vi "24点 - LabVIEW2014 - yuanchgen.vi"() -> ()   [LabVIEW 2014]
uses:
  <vilib>/Utility/file.llb/Read From Spreadsheet File (string).vi
panel:
  out "有解次数":dbl
  in  "重做标志":bool
  in  "重做次数":i32=1
  out "错题库":dbl[][](array[numeric])
  out "time2":dbl=525974.5673637404 caption="相对秒钟" format="%_19f"
  out "time1":dbl=327.1343983679108 caption="相对秒钟" format="%_19f"
  out "time o":dbl=70.42058685328811 caption="相对秒钟" format="%_4f"
  out "开始时间":dbl=525967.1962749355 caption="相对秒钟" format="%_19f"
  out "结束时间":dbl=525974.5673695413 caption="相对秒钟" format="%_19f"
  out "新游戏标志 2":bool
  out "成功次数":dbl=1.0
  out "失败次数":dbl
  in  "新游戏标志":bool
  in  "时间计算标志":bool=TRUE
  out "所有正解":string[](array[string])=["8*(12-9/1)", "8*(12-9)*1"]
  out "算法总数":i32=2
  out "运算符输入次数":dbl
  out "牌值 4":u32=9
  out "牌值 3":u32=1
  out "牌值 2":u32=12
  out "牌值1":u32=8
  in  "游戏界面":enum32{"主界面", "批量计算"}(tab)
  in  "牌遮 3":enum32{"选项卡 1", "选项卡 2"}(tab)
  in  "批量计算":bool=TRUE
  in  "错题重做":bool
  in  "退出游戏":bool=TRUE
  out "已用时间":string="4.04s"
  out "分数提示":string="胜利/失败: 1/0"
  in  "重置":bool
  out "公式显示":string
  in  "牌遮 4":enum32{"选项卡 1", "选项卡 2"}(tab)
  in  "牌遮 2":enum32{"选项卡 1", "选项卡 2"}(tab)
  in  "牌遮 1":enum32{"选项卡 1", "选项卡 2"}(tab)
  out "扑克牌 4":u16(ring)=48
  out "扑克牌 3":u16(ring)=27
  out "扑克牌 2":u16(ring)=51
  out "扑克牌 1":u16(ring)=47
  in  "开始游戏":bool
  in  "偷看答案":bool
  in  "无解":bool
  in  "计算":bool
  in  "右括号":bool
  in  "左括号":bool
  in  "除":bool
  in  "乘":bool
  in  "减":bool
  in  "加":bool
  in  "返回主界面":bool caption="退出游戏"
  out "表格":string[][](table)
  out "结果显示":string="本次批量计算总共完成   组数据，共耗时   s。"
  in  "文件路径输入控件":path
  # "扑克24点"
  # "24点批量计算"
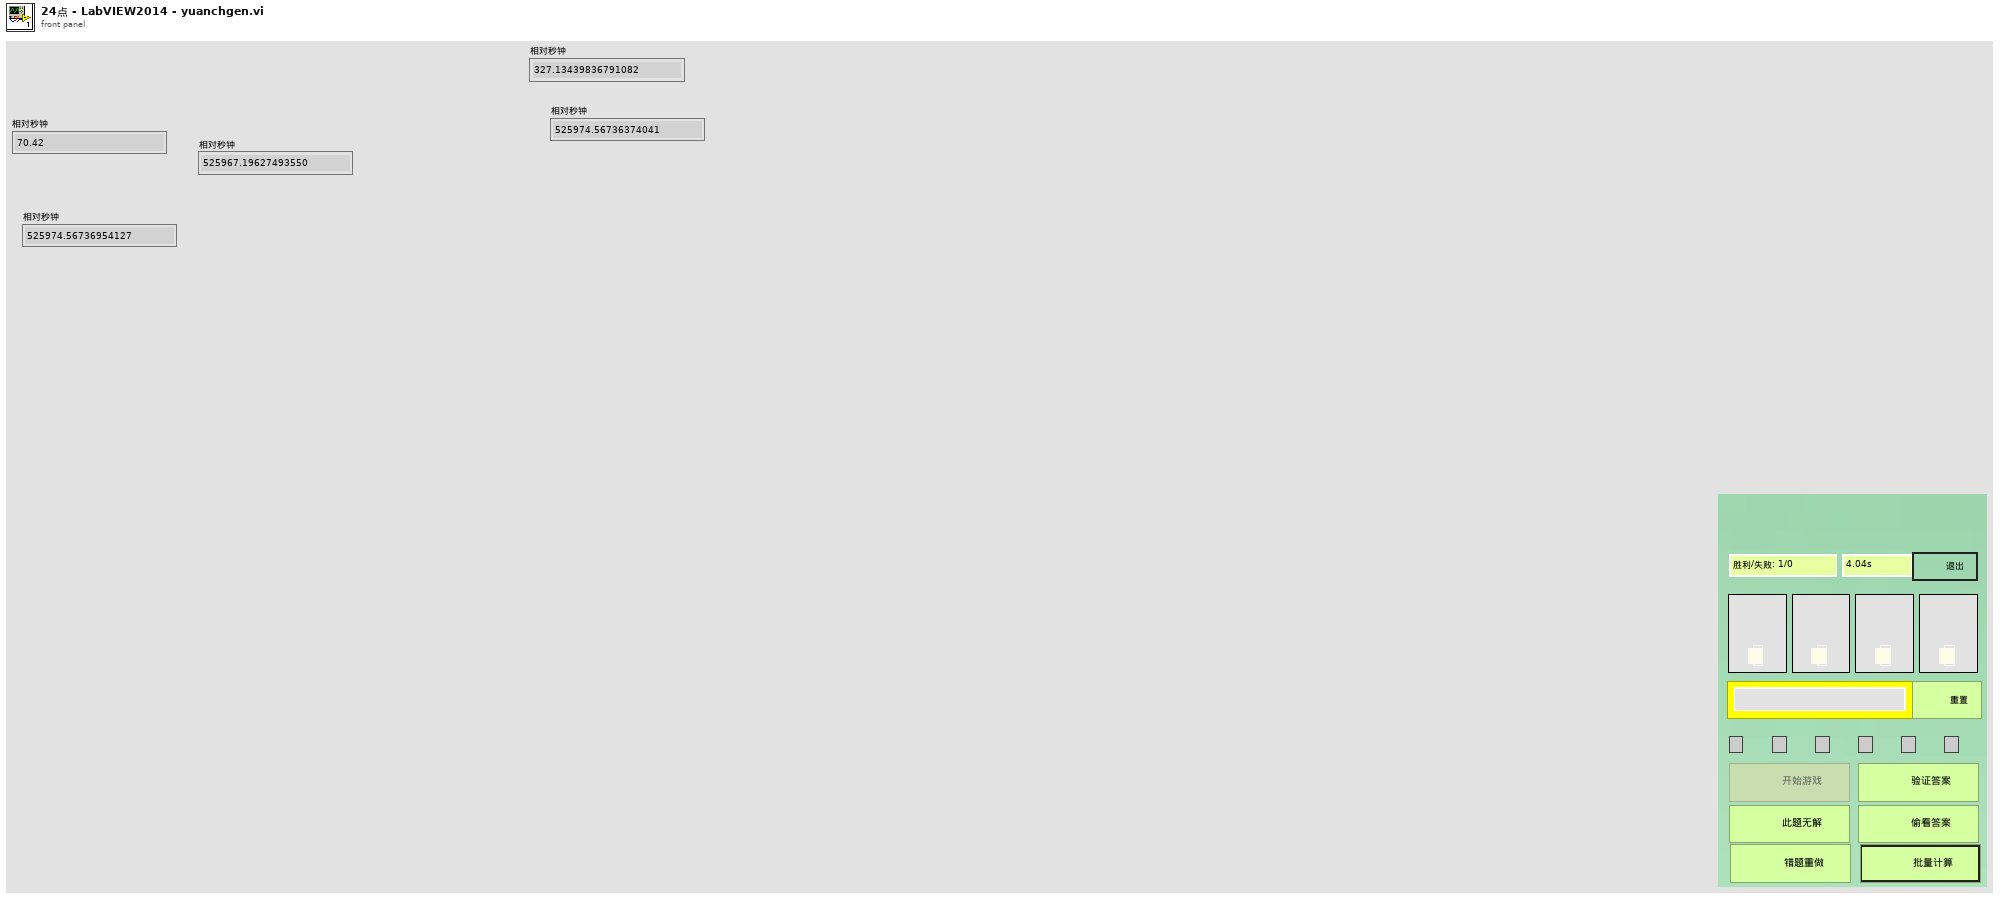
[diagram p1: front panel]
types:
  T1 = enum8{"Enabled", "Disabled", "Disabled and Grayed Out"}
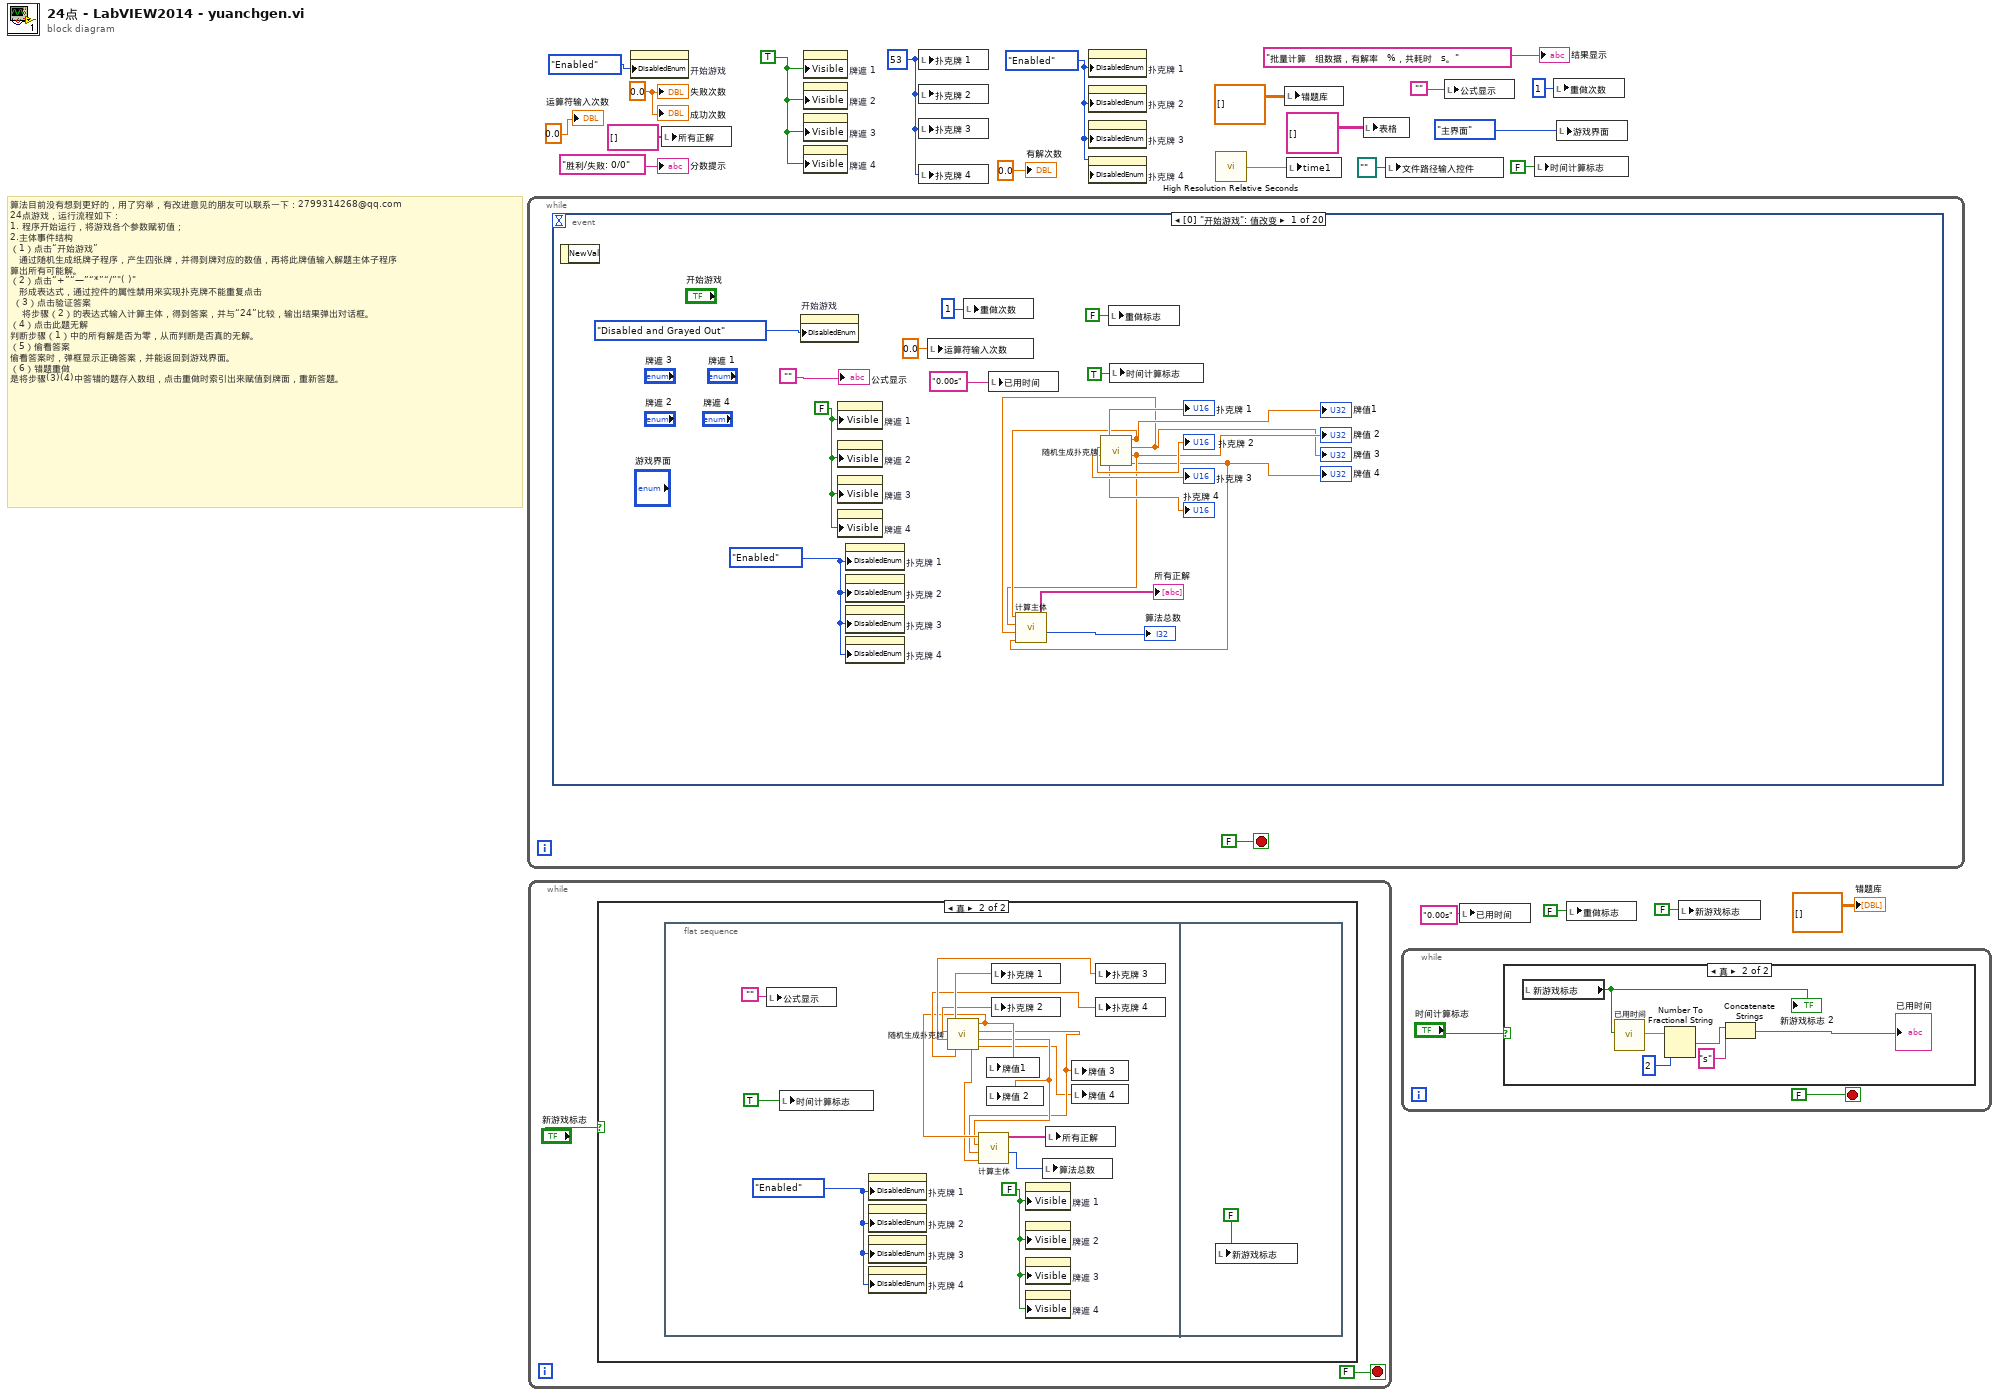
[diagram p0: block diagram]
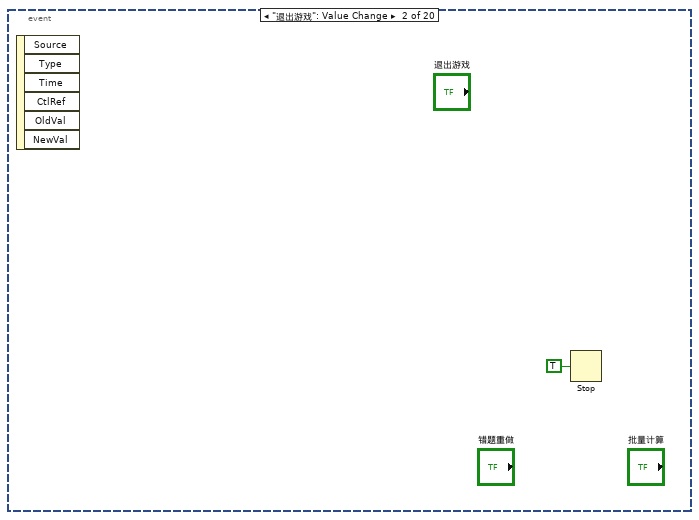
[diagram p4: hidden frame]
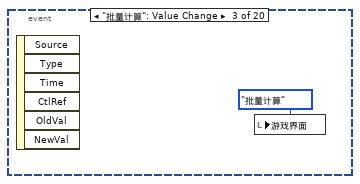
[diagram p5: hidden frame]
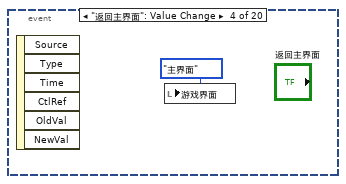
[diagram p6: hidden frame]
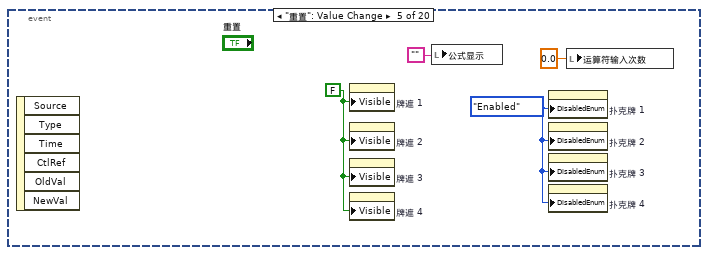
[diagram p7: hidden frame]
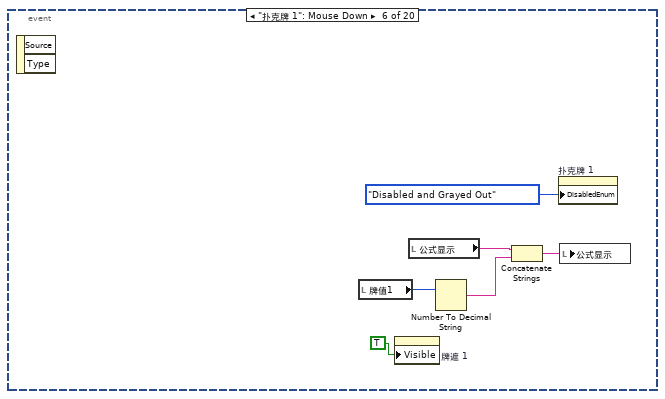
[diagram p8: hidden frame]
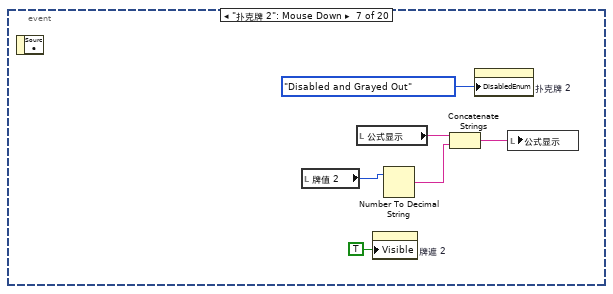
[diagram p9: hidden frame]
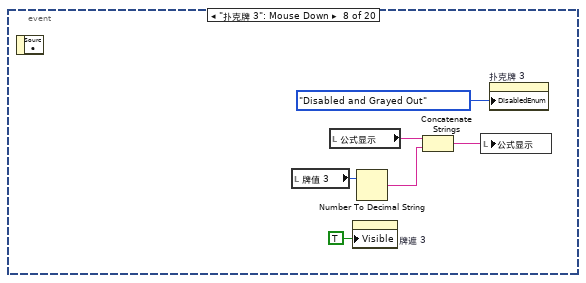
[diagram p10: hidden frame]
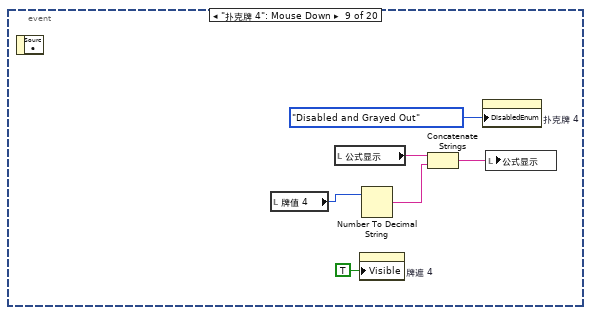
[diagram p11: hidden frame]
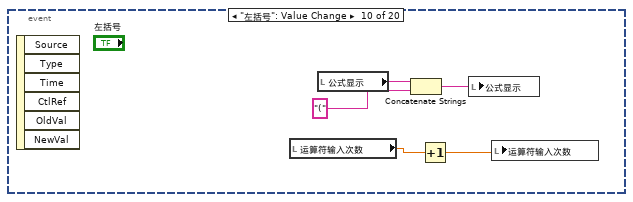
[diagram p12: hidden frame]
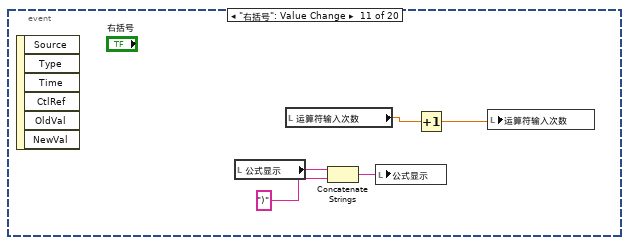
[diagram p13: hidden frame]
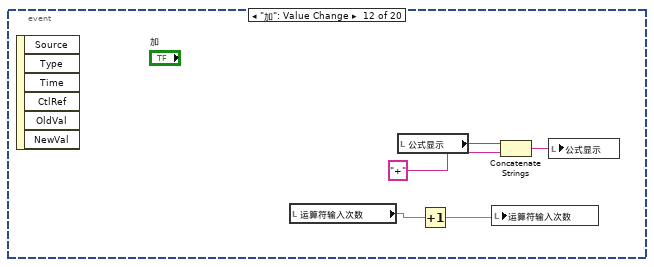
[diagram p14: hidden frame]
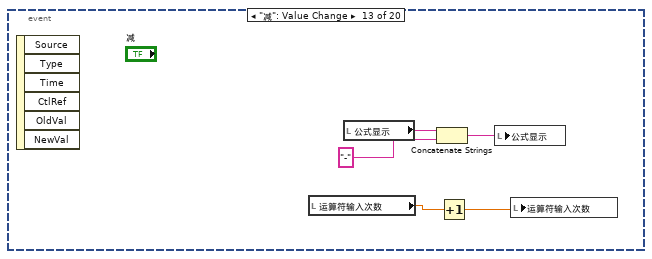
[diagram p15: hidden frame]
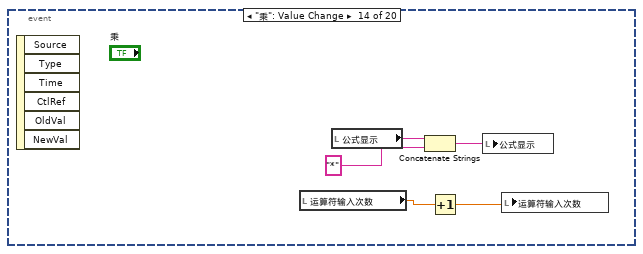
[diagram p16: hidden frame]
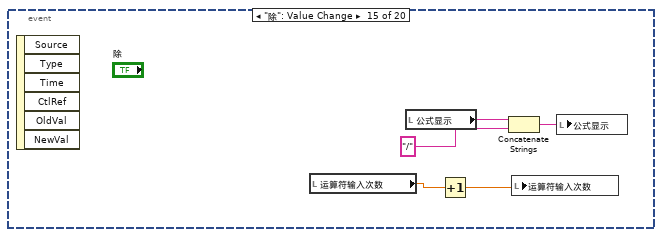
[diagram p17: hidden frame]
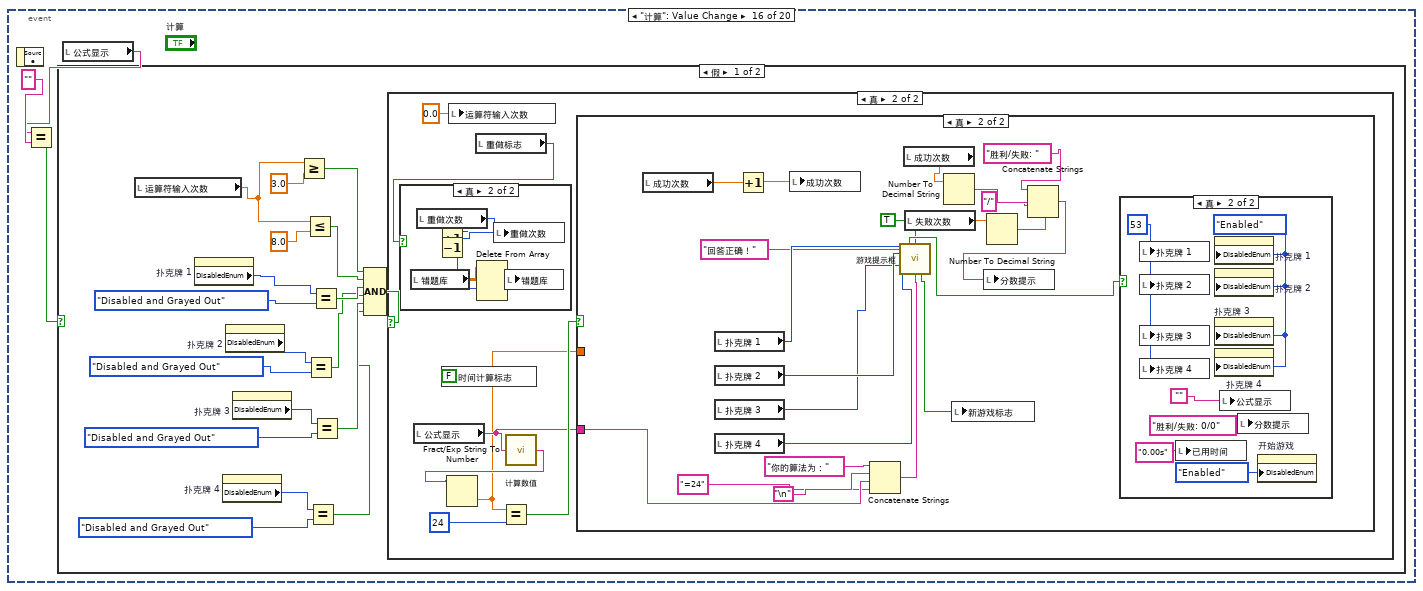
[diagram p18: hidden frame]
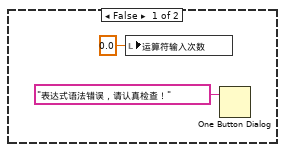
[diagram p19: hidden frame]
diagram:
  w15 = 0.0 ("运算符输入次数 2")
  w20 = TRUE ("可见")
  w21 = T1."Enabled" ("禁用")
  w22 = u16 53 ("扑克牌 1")
  # "算法目前没有想到更好的，用了穷举，有改进意见的朋友可以联系一下：2799314268@qq.com\n24点游戏，运行流程如下：\n1. 程序开始运行，将游戏各个参数赋初值；\n2.主体事件结构\n（1）点击“开始游戏”\n   通过随机生成纸牌子程序，产生四张牌，并得到牌对应的数值，再将此牌值输入解题主体子程序\n算出所有可能解。\n（2）点击“+”“—”“*”“/”\"( )\"\n   形成表达式，通过控件的属性禁用来实现扑克牌不能重复点击\n （3）点击验证答案\n    将步骤（2）的表达式输入计算主体，得到答案，并与“24”比较，输出结果弹出对话框。\n（4）点击此题无解\n判断步骤（1）中的所有解是否为零，从而判断是否真的无解。\n（5）偷看答案\n偷看答案时，弹框显示正确答案，并能返回到游戏界面。\n（6）错题重做\n是将步骤(3)(4)中答错的题存入数组，点击重做时索引出来赋值到牌面，重新答题。"
  n1 = while {
    stop <- FALSE stop-if-true
    n2 = event shown="[0] \"开始游戏\": 值改变" {
      selector: _ -> [_ _ _ _ _ _ _ _ _ _ _ _ _ _ _ _ _ _ _ _]
      dyn-events: _ -> [_ _ _ _ _ _ _ _ _ _ _ _ _ _ _ _ _ _ _ _]
      timeout: _ -> [_ _ _ _ _ _ _ _ _ _ _ _ _ _ _ _ _ _ _ _]
      event "开始游戏": Value Change {
        w40 = FALSE ("可见")
        w42 = T1."Enabled" ("禁用")
        n3 = event-data() -> ()  [unwired: 1 in, 1 out]
        n4 = property on="开始游戏" class="Bool"("DisabledEnum"=T1."Disabled and Grayed Out" ("禁用")) -> ()  [unwired: 2 in, 2 out]
        n5 = property on="牌遮 1" class="TabCtl (严格)"("Visible"=w40) -> ()  [unwired: 2 in, 2 out]
        n6 = property on="牌遮 2" class="TabCtl (严格)"("Visible"=w40) -> ()  [unwired: 2 in, 2 out]
        n7 = property on="牌遮 3" class="TabCtl (严格)"("Visible"=w40) -> ()  [unwired: 2 in, 2 out]
        n8 = property on="牌遮 4" class="TabCtl (严格)"("Visible"=w40) -> ()  [unwired: 2 in, 2 out]
        n9 = property on="扑克牌 1" class="Ring (严格)"("DisabledEnum"=w42) -> ()  [unwired: 2 in, 2 out]
        n10 = property on="扑克牌 2" class="Ring (严格)"("DisabledEnum"=w42) -> ()  [unwired: 2 in, 2 out]
        n11 = property on="扑克牌 3" class="Ring (严格)"("DisabledEnum"=w42) -> ()  [unwired: 2 in, 2 out]
        n12 = property on="扑克牌 4" class="Ring (严格)"("DisabledEnum"=w42) -> ()  [unwired: 2 in, 2 out]
        n13 = local write "运算符输入次数"(0.0 ("运算符输入次数")) -> ()
        n14 = local write "重做次数"(1 ("重做次数")) -> ()
        n15 = local write "已用时间"("0.00s" ("连接的字符串")) -> ()
        n16 = call "随机生成扑克牌.vi"() -> ("牌4值"=w24:dbl, "牌2值"=w26:dbl, "牌3值"=w25:dbl, "牌1值"=w27:dbl, "牌4"=→"扑克牌 4":dbl, "牌3"=→"扑克牌 3":dbl, "牌2"=→"扑克牌 2":dbl, "牌1"=→"扑克牌 1":dbl)
        "牌值1" <- w27
        "牌值 2" <- w26
        "牌值 3" <- w25
        "牌值 4" <- w24
        n17 = call "计算主体.vi"("d"=w24, "c"=w25, "b"=w26, "a"=w27) -> ("算法总数"=→"算法总数":i32, "所有正解"=→"所有正解":string[])  [unwired: 1 in, 1 out]
        n18 = local write "重做标志"(FALSE ("重做标志")) -> ()
        n19 = local write "时间计算标志"(TRUE ("布尔")) -> ()
        "公式显示" <- ""
      }
      event "退出游戏": Value Change {
        n20 = event-data() -> ()  [unwired: 1 in, 6 out]
        n21 = Stop(stop? (T)=TRUE ("停止？(T)")) -> ()
      }
      event "批量计算": Value Change {
        n22 = event-data() -> ()  [unwired: 1 in, 6 out]
        n23 = local write "游戏界面"(enum32{"主界面", "批量计算"}."批量计算" ("选项卡控件")) -> ()
      }
      event "返回主界面": Value Change {
        n24 = event-data() -> ()  [unwired: 1 in, 6 out]
        n25 = local write "游戏界面"(enum32{"主界面", "批量计算"}."主界面" ("选项卡控件")) -> ()
      }
      event "重置": Value Change {
        w47 = T1."Enabled" ("禁用")
        w48 = FALSE ("可见")
        n26 = event-data() -> ()  [unwired: 1 in, 6 out]
        n27 = property on="牌遮 1" class="TabCtl (严格)"("Visible"=w48) -> ()  [unwired: 2 in, 2 out]
        n28 = property on="牌遮 2" class="TabCtl (严格)"("Visible"=w48) -> ()  [unwired: 2 in, 2 out]
        n29 = property on="牌遮 3" class="TabCtl (严格)"("Visible"=w48) -> ()  [unwired: 2 in, 2 out]
        n30 = property on="牌遮 4" class="TabCtl (严格)"("Visible"=w48) -> ()  [unwired: 2 in, 2 out]
        n31 = local write "公式显示"("") -> ()
        n32 = property on="扑克牌 1" class="Ring (严格)"("DisabledEnum"=w47) -> ()  [unwired: 2 in, 2 out]
        n33 = property on="扑克牌 2" class="Ring (严格)"("DisabledEnum"=w47) -> ()  [unwired: 2 in, 2 out]
        n34 = property on="扑克牌 3" class="Ring (严格)"("DisabledEnum"=w47) -> ()  [unwired: 2 in, 2 out]
        n35 = property on="扑克牌 4" class="Ring (严格)"("DisabledEnum"=w47) -> ()  [unwired: 2 in, 2 out]
        n36 = local write "运算符输入次数"(0.0 ("运算符输入次数")) -> ()
      }
      event "扑克牌 1": Mouse Down {
        n37 = event-data() -> ()  [unwired: 1 in, 2 out]
        n38 = local read "牌值1"() -> (w54:u32)
        n39 = property on="牌遮 1" class="TabCtl (严格)"("Visible"=TRUE ("可见")) -> ()  [unwired: 2 in, 2 out]
        n40 = local read "公式显示"() -> (w52:string)
        n41 = Number To Decimal String(number=w54) -> (decimal integer string=w53:string)  [unwired: 1 in]
        n42 = Concatenate Strings(w52, w53) -> (w51:string)
        n43 = property on="扑克牌 1" class="Ring (严格)"("DisabledEnum"=T1."Disabled and Grayed Out" ("禁用")) -> ()  [unwired: 2 in, 2 out]
        n44 = local write "公式显示"(w51) -> ()
      }
      event "扑克牌 2": Mouse Down {
        n45 = event-data() -> ()  [unwired: 1 in, 1 out]
        n46 = local read "牌值 2"() -> (w57:u32)
        n47 = local read "公式显示"() -> (w59:string)
        n48 = property on="牌遮 2" class="TabCtl (严格)"("Visible"=TRUE ("可见")) -> ()  [unwired: 2 in, 2 out]
        n49 = Number To Decimal String(number=w57) -> (decimal integer string=w60:string)  [unwired: 1 in]
        n50 = Concatenate Strings(w59, w60) -> (w58:string)
        n51 = property on="扑克牌 2" class="Ring (严格)"("DisabledEnum"=T1."Disabled and Grayed Out" ("禁用")) -> ()  [unwired: 2 in, 2 out]
        n52 = local write "公式显示"(w58) -> ()
      }
      event "扑克牌 3": Mouse Down {
        n53 = event-data() -> ()  [unwired: 1 in, 1 out]
        n54 = local read "牌值 3"() -> (w63:u32)
        n55 = local read "公式显示"() -> (w66:string)
        n56 = property on="牌遮 3" class="TabCtl (严格)"("Visible"=TRUE ("可见")) -> ()  [unwired: 2 in, 2 out]
        n57 = Number To Decimal String(number=w63) -> (decimal integer string=w64:string)  [unwired: 1 in]
        n58 = Concatenate Strings(w66, w64) -> (w65:string)
        n59 = local write "公式显示"(w65) -> ()
        n60 = property on="扑克牌 3" class="Ring (严格)"("DisabledEnum"=T1."Disabled and Grayed Out" ("禁用")) -> ()  [unwired: 2 in, 2 out]
      }
      event "扑克牌 4": Mouse Down {
        n61 = event-data() -> ()  [unwired: 1 in, 1 out]
        n62 = local read "牌值 4"() -> (w69:u32)
        n63 = local read "公式显示"() -> (w72:string)
        n64 = property on="牌遮 4" class="TabCtl (严格)"("Visible"=TRUE ("可见")) -> ()  [unwired: 2 in, 2 out]
        n65 = Number To Decimal String(number=w69) -> (decimal integer string=w70:string)  [unwired: 1 in]
        n66 = Concatenate Strings(w72, w70) -> (w71:string)
        n67 = property on="扑克牌 4" class="Ring (严格)"("DisabledEnum"=T1."Disabled and Grayed Out" ("禁用")) -> ()  [unwired: 2 in, 2 out]
        n68 = local write "公式显示"(w71) -> ()
      }
      event "左括号": Value Change {
        n69 = event-data() -> ()  [unwired: 1 in, 6 out]
        n70 = local read "运算符输入次数"() -> (w75:dbl)
        n71 = local read "公式显示"() -> (w78:string)
        n72 = Concatenate Strings(w78, "(" ("字符串")) -> (w77:string)
        n73 = Increment(x=w75) -> (x+1=w74:dbl)
        n74 = local write "公式显示"(w77) -> ()
        n75 = local write "运算符输入次数"(w74) -> ()
      }
      event "右括号": Value Change {
        n76 = event-data() -> ()  [unwired: 1 in, 6 out]
        n77 = local read "公式显示"() -> (w83:string)
        n78 = local read "运算符输入次数"() -> (w80:dbl)
        n79 = Concatenate Strings(w83, ")" ("字符串")) -> (w82:string)
        n80 = local write "公式显示"(w82) -> ()
        n81 = Increment(x=w80) -> (x+1=w79:dbl)
        n82 = local write "运算符输入次数"(w79) -> ()
      }
      event "加": Value Change {
        n83 = event-data() -> ()  [unwired: 1 in, 6 out]
        n84 = local read "运算符输入次数"() -> (w85:dbl)
        n85 = local read "公式显示"() -> (w88:string)
        n86 = Increment(x=w85) -> (x+1=w84:dbl)
        n87 = local write "运算符输入次数"(w84) -> ()
        n88 = Concatenate Strings(w88, "+" ("字符串")) -> (w87:string)
        n89 = local write "公式显示"(w87) -> ()
      }
      event "减": Value Change {
        n90 = event-data() -> ()  [unwired: 1 in, 6 out]
        n91 = local read "运算符输入次数"() -> (w90:dbl)
        n92 = local read "公式显示"() -> (w93:string)
        n93 = Concatenate Strings(w93, "-" ("字符串")) -> (w92:string)
        n94 = Increment(x=w90) -> (x+1=w89:dbl)
        n95 = local write "公式显示"(w92) -> ()
        n96 = local write "运算符输入次数"(w89) -> ()
      }
      event "乘": Value Change {
        n97 = event-data() -> ()  [unwired: 1 in, 6 out]
        n98 = local read "运算符输入次数"() -> (w95:dbl)
        n99 = local read "公式显示"() -> (w98:string)
        n100 = Concatenate Strings(w98, "*" ("字符串")) -> (w97:string)
        n101 = Increment(x=w95) -> (x+1=w94:dbl)
        n102 = local write "公式显示"(w97) -> ()
        n103 = local write "运算符输入次数"(w94) -> ()
      }
      event "除": Value Change {
        n104 = event-data() -> ()  [unwired: 1 in, 6 out]
        n105 = local read "运算符输入次数"() -> (w100:dbl)
        n106 = local read "公式显示"() -> (w103:string)
        n107 = Increment(x=w100) -> (x+1=w99:dbl)
        n108 = Concatenate Strings(w103, "/" ("字符串")) -> (w102:string)
        n109 = local write "运算符输入次数"(w99) -> ()
        n110 = local write "公式显示"(w102) -> ()
      }
      event "计算": Value Change {
        n111 = event-data() -> ()  [unwired: 1 in, 1 out]
        n112 = local read "公式显示"() -> (w105:string)
        n113 = Equal?(x=w105, y="" ("公式显示")) -> (x = y?=w104:bool)
        n114 = case shown="假" w104 {
          frame False {
            n115 = local read "运算符输入次数"() -> (w108:dbl)
            n116 = property on="扑克牌 1" class="Ring (严格)"() -> ("DisabledEnum"=w109:T1)  [unwired: 2 in, 2 out]
            n117 = property on="扑克牌 4" class="Ring (严格)"() -> ("DisabledEnum"=w117:T1)  [unwired: 2 in, 2 out]
            n118 = property on="扑克牌 2" class="Ring (严格)"() -> ("DisabledEnum"=w121:T1)  [unwired: 2 in, 2 out]
            n119 = property on="扑克牌 3" class="Ring (严格)"() -> ("DisabledEnum"=w119:T1)  [unwired: 2 in, 2 out]
            n120 = Greater Or Equal?(x=w108, y=3.0) -> (x >= y?=w115:bool)
            n121 = Less Or Equal?(x=w108, y=8.0) -> (x <= y?=w107:bool)
            n122 = Equal?(x=w121, y=T1."Disabled and Grayed Out" ("禁用")) -> (x = y?=w113:bool)
            n123 = Equal?(x=w117, y=T1."Disabled and Grayed Out" ("禁用")) -> (x = y?=w111:bool)
            n124 = Equal?(x=w109, y=T1."Disabled and Grayed Out" ("禁用")) -> (x = y?=w114:bool)
            n125 = Equal?(x=w119, y=T1."Disabled and Grayed Out" ("禁用")) -> (x = y?=w112:bool)
            n126 = Compound Arithmetic op=AND(w115, w107, w114, w113, w112, w111) -> (w110:bool)
            n127 = case shown="真" w110 {
              frame False {
                n128 = local write "运算符输入次数"(0.0 ("运算符输入次数")) -> ()
                n129 = One Button Dialog(message="表达式语法错误，请认真检查！" ("消息")) -> ()  [unwired: 1 in, 1 out]
              }
              frame True {
                n130 = local read "公式显示"() -> (w131:string)
                n131 = local write "时间计算标志"(FALSE ("布尔")) -> ()
                n132 = local write "运算符输入次数"(0.0 ("运算符输入次数")) -> ()
                n133 = local read "重做标志"() -> (w128:bool)
                n134 = case shown="真" w128 {
                  frame False {
                  }
                  frame True {
                    n135 = local read "错题库"() -> (w138:dbl[][])
                    n136 = local read "重做次数"() -> (w135:i32)
                    n137 = Increment(x=w135) -> (x+1=w136:i32)
                    n138 = Decrement(x=w135) -> (x-1=w139:i32)
                    n139 = Delete From Array(array=w138, index (row)=w139) -> (array with subset deleted=w137:dbl[][])  [unwired: 2 in, 1 out]
                    n140 = local write "重做次数"(w136) -> ()
                    n141 = local write "错题库"(w137) -> ()
                  }
                }
                n142 = call "计算数值.vi"("表达式"=w131) -> ("结果"=w132:string)
                n143 = Fract/Exp String To Number(string=w132) -> (number=w130:dbl)  [unwired: 3 in, 1 out]
                n144 = Equal?(x=w130, y=24 ("x")) -> (x = y?=w133:bool)
                n145 = case shown="真" w133 {
                  tunnel: w130 -> [w149 _]
                  tunnel: w131 -> [_ w222]
                  frame False {
                    n146 = local read "成功次数"() -> (w146:dbl)
                    n147 = local read "失败次数"() -> (w142:dbl)
                    n148 = local read "所有正解"() -> (w153:string[])
                    n149 = local read "失败次数"() -> (w148:dbl)
                    n150 = Number To Decimal String(number=w146) -> (decimal integer string=w144:string)  [unwired: 1 in]
                    n151 = Array Size(array=w153) -> (size(s)=w152:i32)
                    n152 = Number To Decimal String(number=w142) -> (decimal integer string=w141:string)  [unwired: 1 in]
                    n153 = Increment(x=w148) -> (x+1=w147:dbl)
                    n154 = local write "失败次数"(w147) -> ()
                    n155 = Equal?(x=0, y=w152) -> (x = y?=w150:bool)
                    n156 = Concatenate Strings("胜利/失败: " ("分数提示"), w144, "/" ("字符串"), w141) -> (w140:string)
                    n157 = local write "分数提示"(w140) -> ()
                    n158 = case shown="真" w150 {
                      tunnel: w149 -> [w174 w199]
                      frame False {
                        n159 = local read "所有正解"() -> (w172:string[])
                        n160 = local read "扑克牌 1"() -> (w159:u16)
                        n161 = local read "扑克牌 2"() -> (w158:u16)
                        n162 = local read "扑克牌 3"() -> (w157:u16)
                        n163 = local read "扑克牌 4"() -> (w156:u16)
                        n164 = Array Size(array=w172) -> (size(s)=w171:i32)
                        n165 = Index Array(array=w172) -> (element=w166:string)  [unwired: 1 in]
                        n166 = Number To Decimal String(number=w171) -> (decimal integer string=w170:string)  [unwired: 1 in]
                        n167 = Number To Decimal String(number=w174) -> (decimal integer string=w177:string)  [unwired: 1 in]
                        n168 = Concatenate Strings("本题有" ("字符串"), w170, "解法！" ("字符串"), "\n", "例如:" ("字符串"), w166, "=24" ("字符串")) -> (w164:string)
                        n169 = Concatenate Strings("回答错误，你的答案为" ("消息"), w177, "！" ("字符串")) -> (w175:string)
                        n170 = call "游戏提示框.vi"("数值1"=w159, "再来一局可见"=TRUE, "结果"=w175, "数值2"=w158, "数值3"=w157, "数值4"=w156, "答案"=w164) -> ("指示灯 2"=w155:bool, "指示灯"=w163:bool)  [unwired: 3 in, 4 out]
                        n171 = local write "新游戏标志"(w163) -> ()
                        n172 = local read "错题库"() -> (w162:dbl[][])
                        n173 = Build Array(w159, w158, w157, w156) -> (w161:u16[])
                        n174 = Build Array (concatenate)(w161, w162) -> (w160:dbl[][])
                        n175 = local write "错题库"(w160) -> ()
                        n176 = case shown="真" w155 {
                          frame False {
                          }
                          frame True {
                            w184 = T1."Enabled" ("禁用")
                            w183 = u16 53 ("扑克牌 1")
                            n177 = local write "扑克牌 1"(w183) -> ()
                            n178 = local write "扑克牌 2"(w183) -> ()
                            n179 = local write "扑克牌 3"(w183) -> ()
                            n180 = local write "扑克牌 4"(w183) -> ()
                            n181 = local write "已用时间"("0.00s" ("连接的字符串")) -> ()
                            n182 = property on="扑克牌 1" class="Ring (严格)"("DisabledEnum"=w184) -> ()  [unwired: 2 in, 2 out]
                            n183 = property on="扑克牌 2" class="Ring (严格)"("DisabledEnum"=w184) -> ()  [unwired: 2 in, 2 out]
                            n184 = property on="扑克牌 3" class="Ring (严格)"("DisabledEnum"=w184) -> ()  [unwired: 2 in, 2 out]
                            n185 = property on="扑克牌 4" class="Ring (严格)"("DisabledEnum"=w184) -> ()  [unwired: 2 in, 2 out]
                            n186 = local write "公式显示"("") -> ()
                            n187 = local write "分数提示"("胜利/失败: 0/0" ("分数提示")) -> ()
                            n188 = property on="开始游戏" class="Bool"("DisabledEnum"=T1."Enabled" ("禁用")) -> ()  [unwired: 2 in, 2 out]
                          }
                        }
                      }
                      frame True {
                        n189 = local read "错题库"() -> (w191:dbl[][])
                        n190 = local read "扑克牌 1"() -> (w190:u16)
                        n191 = local read "扑克牌 2"() -> (w189:u16)
                        n192 = local read "扑克牌 3"() -> (w188:u16)
                        n193 = local read "扑克牌 4"() -> (w187:u16)
                        n194 = Build Array(w190, w189, w188, w187) -> (w192:u16[])
                        n195 = Number To Decimal String(number=w199) -> (decimal integer string=w198:string)  [unwired: 1 in]
                        n196 = Build Array (concatenate)(w192, w191) -> (w193:dbl[][])
                        n197 = local write "错题库"(w193) -> ()
                        n198 = Concatenate Strings("回答错误，你的答案为：" ("消息"), w198, "！" ("字符串")) -> (w196:string)
                        n199 = call "游戏提示框.vi"("数值1"=w190, "再来一局可见"=TRUE, "结果"=w196, "数值2"=w189, "数值3"=w188, "数值4"=w187, "答案"="正确答案：本题无解！") -> ("指示灯 2"=w186:bool, "指示灯"=w194:bool)  [unwired: 3 in, 4 out]
                        n200 = local write "新游戏标志"(w194) -> ()
                        n201 = case shown="真" w186 {
                          frame False {
                          }
                          frame True {
                            w206 = T1."Enabled" ("禁用")
                            w205 = u16 53 ("扑克牌 1")
                            n202 = local write "扑克牌 1"(w205) -> ()
                            n203 = local write "扑克牌 2"(w205) -> ()
                            n204 = local write "扑克牌 3"(w205) -> ()
                            n205 = local write "扑克牌 4"(w205) -> ()
                            n206 = local write "已用时间"("0.00s" ("连接的字符串")) -> ()
                            n207 = property on="扑克牌 1" class="Ring (严格)"("DisabledEnum"=w206) -> ()  [unwired: 2 in, 2 out]
                            n208 = property on="扑克牌 2" class="Ring (严格)"("DisabledEnum"=w206) -> ()  [unwired: 2 in, 2 out]
                            n209 = property on="扑克牌 3" class="Ring (严格)"("DisabledEnum"=w206) -> ()  [unwired: 2 in, 2 out]
                            n210 = property on="扑克牌 4" class="Ring (严格)"("DisabledEnum"=w206) -> ()  [unwired: 2 in, 2 out]
                            n211 = local write "公式显示"("") -> ()
                            n212 = local write "分数提示"("胜利/失败: 0/0" ("分数提示")) -> ()
                            n213 = property on="开始游戏" class="Bool"("DisabledEnum"=T1."Enabled" ("禁用")) -> ()  [unwired: 2 in, 2 out]
                          }
                        }
                      }
                    }
                  }
                  frame True {
                    n214 = local read "成功次数"() -> (w217:dbl)
                    n215 = local read "扑克牌 1"() -> (w228:u16)
                    n216 = local read "扑克牌 2"() -> (w227:u16)
                    n217 = local read "扑克牌 3"() -> (w226:u16)
                    n218 = local read "扑克牌 4"() -> (w225:u16)
                    n219 = Increment(x=w217) -> (x+1=w216:dbl)
                    n220 = local write "成功次数"(w216) -> ()
                    n221 = Concatenate Strings("你的算法为：" ("消息"), "\n", w222, "=24" ("字符串")) -> (w220:string)
                    n222 = call "游戏提示框.vi"("数值1"=w228, "再来一局可见"=TRUE, "结果"="回答正确！" ("消息"), "数值2"=w227, "数值3"=w226, "数值4"=w225, "答案"=w220) -> ("指示灯 2"=w208:bool, "指示灯"=w218:bool)  [unwired: 3 in, 4 out]
                    n223 = local read "成功次数"() -> (w215:dbl)
                    n224 = local read "失败次数"() -> (w212:dbl)
                    n225 = Number To Decimal String(number=w215) -> (decimal integer string=w214:string)  [unwired: 1 in]
                    n226 = local write "新游戏标志"(w218) -> ()
                    n227 = Number To Decimal String(number=w212) -> (decimal integer string=w211:string)  [unwired: 1 in]
                    n228 = Concatenate Strings("胜利/失败: " ("分数提示"), w214, "/" ("字符串"), w211) -> (w209:string)
                    n229 = local write "分数提示"(w209) -> ()
                    n230 = case shown="真" w208 {
                      frame False {
                      }
                      frame True {
                        w234 = T1."Enabled" ("禁用")
                        w233 = u16 53 ("扑克牌 1")
                        n231 = local write "扑克牌 1"(w233) -> ()
                        n232 = local write "扑克牌 2"(w233) -> ()
                        n233 = local write "扑克牌 3"(w233) -> ()
                        n234 = local write "扑克牌 4"(w233) -> ()
                        n235 = local write "已用时间"("0.00s" ("连接的字符串")) -> ()
                        n236 = property on="扑克牌 1" class="Ring (严格)"("DisabledEnum"=w234) -> ()  [unwired: 2 in, 2 out]
                        n237 = property on="扑克牌 2" class="Ring (严格)"("DisabledEnum"=w234) -> ()  [unwired: 2 in, 2 out]
                        n238 = property on="扑克牌 3" class="Ring (严格)"("DisabledEnum"=w234) -> ()  [unwired: 2 in, 2 out]
                        n239 = property on="扑克牌 4" class="Ring (严格)"("DisabledEnum"=w234) -> ()  [unwired: 2 in, 2 out]
                        n240 = local write "公式显示"("") -> ()
                        n241 = local write "分数提示"("胜利/失败: 0/0" ("分数提示")) -> ()
                        n242 = property on="开始游戏" class="Bool"("DisabledEnum"=T1."Enabled" ("禁用")) -> ()  [unwired: 2 in, 2 out]
                      }
                    }
                  }
                }
              }
            }
          }
          frame True {
            n243 = One Button Dialog(message="表达式不能为空！" ("消息")) -> ()  [unwired: 1 in, 1 out]
          }
        }
      }
      event "无解": Value Change {
        n244 = event-data() -> ()  [unwired: 1 in, 1 out]
        n245 = local read "扑克牌 1"() -> (w238:u16)
        n246 = Equal?(x=w238, y=u16 53 ("扑克牌 1")) -> (x = y?=w236:bool)
        n247 = case shown="假" w236 {
          frame False {
            n248 = local read "所有正解"() -> (w243:string[])
            n249 = Array Size(array=w243) -> (size(s)=w242:i32)
            n250 = local write "时间计算标志"(FALSE ("布尔")) -> ()
            n251 = Equal?(x=0, y=w242) -> (x = y?=w240:bool)
            n252 = case shown="假" w240 {
              frame False {
                n253 = local read "所有正解"() -> (w272:string[])
                n254 = Array Size(array=w272) -> (size(s)=w271:i32)
                n255 = Index Array(array=w272) -> (element=w266:string)  [unwired: 1 in]
                n256 = Number To Decimal String(number=w271) -> (decimal integer string=w270:string)  [unwired: 1 in]
                n257 = local read "失败次数"() -> (w262:dbl)
                n258 = local read "扑克牌 1"() -> (w251:u16)
                n259 = local read "扑克牌 2"() -> (w250:u16)
                n260 = local read "扑克牌 3"() -> (w249:u16)
                n261 = local read "扑克牌 4"() -> (w248:u16)
                n262 = Increment(x=w262) -> (x+1=w261:dbl)
                n263 = local write "失败次数"(w261) -> ()
                n264 = Concatenate Strings("本题有" ("字符串"), w270, "解法！" ("字符串"), "\n", "例如:" ("字符串"), w266, "=24" ("字符串")) -> (w265:string)
                n265 = local read "重做标志"() -> (w246:bool)
                n266 = call "游戏提示框.vi"("数值1"=w251, "再来一局可见"=TRUE, "结果"="回答错误！", "数值2"=w250, "数值3"=w249, "数值4"=w248, "答案"=w265) -> ("指示灯 2"=w245:bool, "指示灯"=w263:bool)  [unwired: 3 in, 4 out]
                n267 = case shown="真" w246 {
                  frame False {
                  }
                  frame True {
                    n268 = local read "错题库"() -> (w284:dbl[][])
                    n269 = local read "重做次数"() -> (w283:i32)
                    n270 = Decrement(x=w283) -> (x-1=w285:i32)
                    n271 = Delete From Array(array=w284, index (row)=w285) -> (array with subset deleted=w281:dbl[][])  [unwired: 2 in, 1 out]
                    n272 = Increment(x=w283) -> (x+1=w282:i32)
                    n273 = local write "重做次数"(w282) -> ()
                    n274 = local write "错题库"(w281) -> ()
                  }
                }
                n275 = local write "新游戏标志"(w263) -> ()
                n276 = local read "成功次数"() -> (w254:dbl)
                n277 = local read "失败次数"() -> (w258:dbl)
                n278 = local read "错题库"() -> (w247:dbl[][])
                n279 = Build Array(w251, w250, w249, w248) -> (w252:u16[])
                n280 = Number To Decimal String(number=w254) -> (decimal integer string=w260:string)  [unwired: 1 in]
                n281 = Build Array (concatenate)(w252, w247) -> (w253:dbl[][])
                n282 = Number To Decimal String(number=w258) -> (decimal integer string=w257:string)  [unwired: 1 in]
                n283 = local write "错题库"(w253) -> ()
                n284 = Concatenate Strings("胜利/失败: " ("分数提示"), w260, "/" ("字符串"), w257) -> (w255:string)
                n285 = local write "分数提示"(w255) -> ()
                n286 = case shown="真" w245 {
                  frame False {
                  }
                  frame True {
                    w280 = T1."Enabled" ("禁用")
                    w279 = u16 53 ("扑克牌 1")
                    n287 = local write "扑克牌 1"(w279) -> ()
                    n288 = local write "扑克牌 2"(w279) -> ()
                    n289 = local write "扑克牌 3"(w279) -> ()
                    n290 = local write "扑克牌 4"(w279) -> ()
                    n291 = local write "已用时间"("0.00s" ("连接的字符串")) -> ()
                    n292 = property on="扑克牌 1" class="Ring (严格)"("DisabledEnum"=w280) -> ()  [unwired: 2 in, 2 out]
                    n293 = property on="扑克牌 2" class="Ring (严格)"("DisabledEnum"=w280) -> ()  [unwired: 2 in, 2 out]
                    n294 = property on="扑克牌 3" class="Ring (严格)"("DisabledEnum"=w280) -> ()  [unwired: 2 in, 2 out]
                    n295 = property on="扑克牌 4" class="Ring (严格)"("DisabledEnum"=w280) -> ()  [unwired: 2 in, 2 out]
                    n296 = local write "公式显示"("") -> ()
                    n297 = local write "分数提示"("胜利/失败: 0/0" ("分数提示")) -> ()
                    n298 = property on="开始游戏" class="Bool"("DisabledEnum"=T1."Enabled" ("禁用")) -> ()  [unwired: 2 in, 2 out]
                  }
                }
              }
              frame True {
                n299 = local read "扑克牌 1"() -> (w302:u16)
                n300 = local read "扑克牌 2"() -> (w301:u16)
                n301 = local read "扑克牌 3"() -> (w300:u16)
                n302 = local read "扑克牌 4"() -> (w299:u16)
                n303 = local read "成功次数"() -> (w297:dbl)
                n304 = Increment(x=w297) -> (x+1=w296:dbl)
                n305 = local write "成功次数"(w296) -> ()
                n306 = call "游戏提示框.vi"("数值1"=w302, "再来一局可见"=TRUE, "结果"="回答正确！" ("消息"), "数值2"=w301, "数值3"=w300, "数值4"=w299, "答案"="本题无解！") -> ("指示灯 2"=w287:bool, "指示灯"=w298:bool)  [unwired: 3 in, 4 out]
                n307 = local read "成功次数"() -> (w289:dbl)
                n308 = local read "失败次数"() -> (w293:dbl)
                n309 = Number To Decimal String(number=w289) -> (decimal integer string=w295:string)  [unwired: 1 in]
                n310 = case shown="真" "重做标志" {
                  frame False {
                  }
                  frame True {
                    n311 = local read "错题库"() -> (w314:dbl[][])
                    n312 = local read "重做次数"() -> (w313:i32)
                    n313 = Decrement(x=w313) -> (x-1=w315:i32)
                    n314 = Delete From Array(array=w314, index (row)=w315) -> (array with subset deleted=w311:dbl[][])  [unwired: 2 in, 1 out]
                    n315 = Increment(x=w313) -> (x+1=w312:i32)
                    n316 = local write "重做次数"(w312) -> ()
                    n317 = local write "错题库"(w311) -> ()
                  }
                }
                n318 = local write "新游戏标志"(w298) -> ()
                n319 = Number To Decimal String(number=w293) -> (decimal integer string=w292:string)  [unwired: 1 in]
                n320 = Concatenate Strings("胜利/失败: " ("分数提示"), w295, "/" ("字符串"), w292) -> (w290:string)
                n321 = local write "分数提示"(w290) -> ()
                n322 = case shown="真" w287 {
                  frame False {
                  }
                  frame True {
                    w310 = T1."Enabled" ("禁用")
                    w309 = u16 53 ("扑克牌 1")
                    n323 = local write "扑克牌 1"(w309) -> ()
                    n324 = local write "扑克牌 2"(w309) -> ()
                    n325 = local write "扑克牌 3"(w309) -> ()
                    n326 = local write "扑克牌 4"(w309) -> ()
                    n327 = local write "已用时间"("0.00s" ("连接的字符串")) -> ()
                    n328 = property on="扑克牌 1" class="Ring (严格)"("DisabledEnum"=w310) -> ()  [unwired: 2 in, 2 out]
                    n329 = property on="扑克牌 2" class="Ring (严格)"("DisabledEnum"=w310) -> ()  [unwired: 2 in, 2 out]
                    n330 = property on="扑克牌 3" class="Ring (严格)"("DisabledEnum"=w310) -> ()  [unwired: 2 in, 2 out]
                    n331 = property on="扑克牌 4" class="Ring (严格)"("DisabledEnum"=w310) -> ()  [unwired: 2 in, 2 out]
                    n332 = local write "公式显示"("") -> ()
                    n333 = local write "分数提示"("胜利/失败: 0/0" ("分数提示")) -> ()
                    n334 = property on="开始游戏" class="Bool"("DisabledEnum"=T1."Enabled" ("禁用")) -> ()  [unwired: 2 in, 2 out]
                  }
                }
              }
            }
          }
          frame True {
            n335 = One Button Dialog(message="请先翻拍！" ("消息")) -> ()  [unwired: 1 in, 1 out]
          }
        }
      }
      event "偷看答案": Value Change {
        n336 = event-data() -> ()  [unwired: 1 in, 1 out]
        n337 = local read "扑克牌 1"() -> (w319:u16)
        n338 = Equal?(x=w319, y=u16 53 ("扑克牌 1")) -> (x = y?=w317:bool)
        n339 = case shown="假" w317 {
          frame False {
            n340 = local read "所有正解"() -> (w324:string[])
            n341 = local write "时间计算标志"(FALSE ("布尔")) -> ()
            n342 = Array Size(array=w324) -> (size(s)=w323:i32)
            n343 = Equal?(x=0, y=w323) -> (x = y?=w321:bool)
            n344 = case shown="真" w321 {
              frame False {
                n345 = local read "所有正解"() -> (w341:string[])
                n346 = Array Size(array=w341) -> (size(s)=w340:i32)
                n347 = Index Array(array=w341) -> (element=w335:string)  [unwired: 1 in]
                n348 = Number To Decimal String(number=w340) -> (decimal integer string=w339:string)  [unwired: 1 in]
                n349 = local read "扑克牌 1"() -> (w333:u16)
                n350 = local read "扑克牌 2"() -> (w332:u16)
                n351 = local read "扑克牌 3"() -> (w331:u16)
                n352 = local read "扑克牌 4"() -> (w330:u16)
                n353 = Concatenate Strings("本题有" ("字符串"), w339, "解法！" ("字符串"), "\n", "例如:" ("字符串"), w335, "=24" ("字符串")) -> (w334:string)
                n354 = call "游戏提示框.vi"("数值1"=w333, "结果"="此题尚未作答！", "数值2"=w332, "数值3"=w331, "数值4"=w330, "返回游戏可见"=TRUE, "答案"=w334) -> ("指示灯 2"=w326:bool, "指示灯"=w328:bool)  [unwired: 3 in, 4 out]
                n355 = local write "新游戏标志"(w328) -> ()
                n356 = case shown="真" w326 {
                  frame False {
                  }
                  frame True {
                    w348 = T1."Enabled" ("禁用")
                    w347 = u16 53 ("扑克牌 1")
                    n357 = local write "扑克牌 1"(w347) -> ()
                    n358 = local write "扑克牌 2"(w347) -> ()
                    n359 = local write "扑克牌 3"(w347) -> ()
                    n360 = local write "扑克牌 4"(w347) -> ()
                    n361 = local write "已用时间"("0.00s" ("连接的字符串")) -> ()
                    n362 = property on="扑克牌 1" class="Ring (严格)"("DisabledEnum"=w348) -> ()  [unwired: 2 in, 2 out]
                    n363 = property on="扑克牌 2" class="Ring (严格)"("DisabledEnum"=w348) -> ()  [unwired: 2 in, 2 out]
                    n364 = property on="扑克牌 3" class="Ring (严格)"("DisabledEnum"=w348) -> ()  [unwired: 2 in, 2 out]
                    n365 = property on="扑克牌 4" class="Ring (严格)"("DisabledEnum"=w348) -> ()  [unwired: 2 in, 2 out]
                    n366 = local write "公式显示"("") -> ()
                    n367 = local write "分数提示"("胜利/失败: 0/0" ("分数提示")) -> ()
                    n368 = property on="开始游戏" class="Bool"("DisabledEnum"=T1."Enabled" ("禁用")) -> ()  [unwired: 2 in, 2 out]
                  }
                }
              }
              frame True {
                n369 = local read "扑克牌 1"() -> (w356:u16)
                n370 = local read "扑克牌 2"() -> (w355:u16)
                n371 = local read "扑克牌 3"() -> (w354:u16)
                n372 = local read "扑克牌 4"() -> (w352:u16)
                n373 = call "游戏提示框.vi"("数值1"=w356, "结果"="此题尚未作答\n本题无解！" ("消息"), "数值2"=w355, "数值3"=w354, "数值4"=w352, "返回游戏可见"=TRUE) -> ("指示灯 2"=w349:bool, "指示灯"=w351:bool)  [unwired: 4 in, 4 out]
                n374 = local write "新游戏标志"(w351) -> ()
                n375 = case shown="真" w349 {
                  frame False {
                  }
                  frame True {
                    w362 = T1."Enabled" ("禁用")
                    w361 = u16 53 ("扑克牌 1")
                    n376 = local write "扑克牌 1"(w361) -> ()
                    n377 = local write "扑克牌 2"(w361) -> ()
                    n378 = local write "扑克牌 3"(w361) -> ()
                    n379 = local write "扑克牌 4"(w361) -> ()
                    n380 = local write "已用时间"("0.00s" ("连接的字符串")) -> ()
                    n381 = property on="扑克牌 1" class="Ring (严格)"("DisabledEnum"=w362) -> ()  [unwired: 2 in, 2 out]
                    n382 = property on="扑克牌 2" class="Ring (严格)"("DisabledEnum"=w362) -> ()  [unwired: 2 in, 2 out]
                    n383 = property on="扑克牌 3" class="Ring (严格)"("DisabledEnum"=w362) -> ()  [unwired: 2 in, 2 out]
                    n384 = property on="扑克牌 4" class="Ring (严格)"("DisabledEnum"=w362) -> ()  [unwired: 2 in, 2 out]
                    n385 = local write "公式显示"("") -> ()
                    n386 = local write "分数提示"("胜利/失败: 0/0" ("分数提示")) -> ()
                    n387 = property on="开始游戏" class="Bool"("DisabledEnum"=T1."Enabled" ("禁用")) -> ()  [unwired: 2 in, 2 out]
                  }
                }
              }
            }
          }
          frame True {
            n388 = One Button Dialog(message="请先翻拍！" ("消息")) -> ()  [unwired: 1 in, 1 out]
          }
        }
      }
      event "文件路径输入控件": Value Change {
        n389 = event-data() -> ()  [unwired: 1 in, 1 out]
        n390 = call-poly <vilib>:"Read From Spreadsheet File.vi"("file path (dialog if empty)"="文件路径输入控件") -> ("all rows"=w370:string[][])  [unwired: 6 in, 4 out]
        n391 = local write "结果显示"("批量计算   组数据，有解率   %，共耗时   s。" ("字符串")) -> ()
        n392 = local write "表格"(string[][] [] ("表格")) -> ()
        n393 = local write "有解次数"(0.0 ("无解次数")) -> ()
        n394 = Array Size(array=w370) -> (size(s)=w368:i32[])
        n395 = Index Array(array=w368) -> (element=w369:i32)  [unwired: 1 in]
        n396 = for {
          N: w369 -> [w371]
          tunnel: w370 -> [w387] mode=indexing
          i -> [w376]
          n397 = Quotient & Remainder(x=w376, y=2) -> (x-y*floor(x/y)=w400:i32)  [unwired: 1 out]
          n398 = Index Array(array=w387) -> (element=w374:string)  [unwired: 1 in]
          n399 = Equal?(x=w376, y=0) -> (x = y?=w393:bool)
          n400 = Decrement(x=w371) -> (x-1=w382:i32)
          n401 = Equal?(x=w400, y=1) -> (x = y?=w402:bool)
          n402 = Match Pattern(string=w374, regular expression="," ("正则表达式")) -> (before substring=w412:string, after substring=w417:string)  [unwired: 1 in, 2 out]
          n403 = Select(t=TRUE, s=w402, f=FALSE) -> (s? t:f=w383:bool)
          n404 = Equal?(x=w376, y=w382) -> (x = y?=w392:bool)
          n405 = Decimal String To Number(string=w412) -> (number=w381:i32)  [unwired: 2 in, 1 out]
          n406 = case shown="真" w392 {
            selector: w392 -> [_ w419]
            tunnel: [_ w419] -> w372
            frame False {
            }
            frame True {
              n407 = call <vilib>:"High Resolution Relative Seconds.vi"() -> ("relative seconds"=→"结束时间":dbl)
            }
          }
          n408 = case shown="真" w393 {
            frame False {
            }
            frame True {
              n409 = call <vilib>:"High Resolution Relative Seconds.vi"() -> ("relative seconds"=→"开始时间":dbl)
            }
          }
          n410 = case shown="真" w383 {
            frame False {
              n411 = call <vilib>:"High Resolution Relative Seconds.vi"() -> ("relative seconds"=w442:dbl)
              "time1" <- w442
              n412 = local read "time2"() -> (w447:dbl)
              n413 = Subtract(x=w447, y=w442) -> (x-y=w446:dbl)
              n414 = Absolute Value(x=w446) -> (abs(x)=w445:dbl)
              n415 = Multiply(x=w445, y=1000.0) -> (x*y=→"time o":dbl)
            }
            frame True {
              n416 = call <vilib>:"High Resolution Relative Seconds.vi"() -> ("relative seconds"=w448:dbl)
              "time2" <- w448
              n417 = local read "time1"() -> (w453:dbl)
              n418 = Subtract(x=w453, y=w448) -> (x-y=w452:dbl)
              n419 = Absolute Value(x=w452) -> (abs(x)=w451:dbl)
              n420 = Multiply(x=w451, y=1000.0) -> (x*y=w449:dbl)
              n421 = local write "time o"(w449) -> ()
            }
          }
          n422 = Match Pattern(string=w417, regular expression="," ("正则表达式")) -> (before substring=w411:string, after substring=w415:string)  [unwired: 1 in, 2 out]
          n423 = Decimal String To Number(string=w411) -> (number=w386:i32)  [unwired: 2 in, 1 out]
          n424 = Match Pattern(string=w415, regular expression="," ("正则表达式")) -> (before substring=w385:string, after substring=w384:string)  [unwired: 1 in, 2 out]
          n425 = Decimal String To Number(string=w385) -> (number=w380:i32)  [unwired: 2 in, 1 out]
          n426 = Match Pattern(string=w384, regular expression="," ("正则表达式")) -> (before substring=w410:string)  [unwired: 1 in, 3 out]
          n427 = Decimal String To Number(string=w410) -> (number=w379:i32)  [unwired: 2 in, 1 out]
          n428 = call "计算主体.vi"("d"=w379, "c"=w380, "b"=w386, "a"=w381) -> ("连接的字符串"=w378:string, "算法总数"=w405:i32)  [unwired: 1 in, 1 out]
          n429 = Equal?(x=0, y=w405) -> (x = y?=w406:bool)
          n430 = local read "time o"() -> (w398:dbl)
          n431 = Increment(x=w376) -> (x+1=w391:i32)
          n432 = Number To Decimal String(number=w405) -> (decimal integer string=w409:string)  [unwired: 1 in]
          n433 = case shown="假" w406 {
            tunnel: w378 -> [w456 _]
            tunnel: [w456 "本题无解" ("连接的字符串")] -> w396
            frame False {
              n434 = local read "有解次数"() -> (w455:dbl)
              n435 = Increment(x=w455) -> (x+1=w454:dbl)
              n436 = local write "有解次数"(w454) -> ()
            }
            frame True {
            }
          }
          n437 = Concatenate Strings(w409, "种" ("字符串")) -> (w407:string)
          n438 = Number To Fractional String(number=w398, precision (6)=i16 2 ("精度(6)")) -> (F-format string=w397:string)  [unwired: 2 in]
          n439 = Number To Fractional String(number=w391, precision (6)=i16 0 ("精度(6)")) -> (F-format string=w375:string)  [unwired: 2 in]
          n440 = case shown="真" w372 {
            tunnel: w371 -> [_ w424]
            frame False {
            }
            frame True {
              n441 = local read "结束时间"() -> (w440:dbl)
              n442 = local read "开始时间"() -> (w441:dbl)
              n443 = local read "有解次数"() -> (w435:dbl)
              n444 = Number To Fractional String(number=w424, precision (6)=i16 0 ("精度(6)")) -> (F-format string=w430:string)  [unwired: 2 in]
              n445 = Wait (ms)(milliseconds to wait=u32 200 ("等待时间（毫秒）")) -> ()  [unwired: 1 out]
              n446 = Subtract(x=w440, y=w441) -> (x-y=w439:dbl)
              n447 = Multiply(x=w435, y=100.0) -> (x*y=w433:dbl)
              n448 = Divide(x=w433, y=w424) -> (x/y=w432:dbl)
              n449 = Number To Fractional String(number=w439, precision (6)=i16 2 ("精度(6)")) -> (F-format string=w426:string)  [unwired: 2 in]
              n450 = Number To Fractional String(number=w432, precision (6)=i16 2 ("精度(6)")) -> (F-format string=w428:string)  [unwired: 2 in]
              n451 = Concatenate Strings("批量计算" ("字符串"), w430, "组数据,有解率" ("字符串"), w428, "%,共耗时" ("字符串"), w426, "s。" ("字符串")) -> (w437:string)
              n452 = local write "结果显示"(w437) -> ()
            }
          }
          n453 = local read "表格"() -> (w388:string[][])
          n454 = Build Array(w375, w374, w407, w397, w396) -> (w389:string[])
          n455 = Build Array (concatenate)(w389, w388) -> (→"表格":string[][])
        }
      }
      event "错题重做": Value Change {
        n456 = event-data() -> ()  [unwired: 1 in, 1 out]
        n457 = local read "失败次数"() -> (w458:dbl)
        n458 = Equal?(x=w458, y=0.0) -> (x = y?=w459:bool)
        n459 = case shown="假" w459 {
          tunnel: w458 -> [w462 _]
          frame False {
            n460 = local read "重做次数"() -> (w463:i32)
            n461 = Less Or Equal?(x=w463, y=w462) -> (x <= y?=w461:bool)
            n462 = case shown="真" w461 {
              frame False {
                n463 = One Button Dialog(message="错题已全部做完！" ("消息")) -> ()  [unwired: 1 in, 1 out]
              }
              frame True {
                w465 = T1."Enabled" ("禁用")
                w484 = FALSE ("可见")
                n464 = local read "错题库"() -> (w468:dbl[][])
                n465 = local write "重做标志"(TRUE ("重做标志")) -> ()
                n466 = local write "公式显示"("") -> ()
                n467 = property on="扑克牌 1" class="Ring (严格)"("DisabledEnum"=w465) -> ()  [unwired: 2 in, 2 out]
                n468 = property on="扑克牌 2" class="Ring (严格)"("DisabledEnum"=w465) -> ()  [unwired: 2 in, 2 out]
                n469 = property on="扑克牌 3" class="Ring (严格)"("DisabledEnum"=w465) -> ()  [unwired: 2 in, 2 out]
                n470 = property on="扑克牌 4" class="Ring (严格)"("DisabledEnum"=w465) -> ()  [unwired: 2 in, 2 out]
                n471 = property on="牌遮 1" class="TabCtl (严格)"("Visible"=w484) -> ()  [unwired: 2 in, 2 out]
                n472 = property on="牌遮 2" class="TabCtl (严格)"("Visible"=w484) -> ()  [unwired: 2 in, 2 out]
                n473 = property on="牌遮 3" class="TabCtl (严格)"("Visible"=w484) -> ()  [unwired: 2 in, 2 out]
                n474 = property on="牌遮 4" class="TabCtl (严格)"("Visible"=w484) -> ()  [unwired: 2 in, 2 out]
                n475 = Decrement(x="重做次数") -> (x-1=w467:i32)
                n476 = Index Array(array=w468, index (row)=w467, index (col)=w467) -> (element=w476:dbl)
                n477 = Index Array(array=w468, index (row)=w467, index (col)=1 ("禁用的索引 (列)")) -> (element=w475:dbl)
                n478 = Index Array(array=w468, index (row)=w467, index (col)=2 ("禁用的索引 (列)")) -> (element=w474:dbl)
                n479 = Index Array(array=w468, index (row)=w467, index (col)=3 ("禁用的索引 (列)")) -> (element=w473:dbl)
                n480 = local write "扑克牌 1"(w476) -> ()
                n481 = local write "扑克牌 2"(w475) -> ()
                n482 = call "得出牌值.vi"("牌4"=w473, "牌3"=w474, "牌2"=w475, "牌1"=w476) -> ("牌4值"=w469:dbl, "牌2值"=w471:dbl, "牌3值"=w470:dbl, "牌1值"=w472:dbl)
                n483 = call "计算主体.vi"("d"=w469, "c"=w470, "b"=w471, "a"=w472) -> ("算法总数"=w483:i32, "所有正解"=w482:string[])  [unwired: 1 in, 1 out]
                n484 = local write "扑克牌 3"(w474) -> ()
                n485 = local write "扑克牌 4"(w473) -> ()
                n486 = local write "算法总数"(w483) -> ()
                n487 = local write "所有正解"(w482) -> ()
                n488 = local write "牌值1"(w472) -> ()
                n489 = local write "牌值 2"(w471) -> ()
                n490 = local write "牌值 3"(w470) -> ()
                n491 = local write "牌值 4"(w469) -> ()
              }
            }
          }
          frame True {
            n492 = One Button Dialog(message="你还没有错题记录！" ("消息")) -> ()  [unwired: 1 in, 1 out]
          }
        }
      }
    }
  }
  n493 = while {
    stop <- FALSE stop-if-true
    n494 = case shown="真" "新游戏标志" {
      frame False {
      }
      frame True {
        n495 = flat-sequence {
          frame #0 {
            w497 = T1."Enabled" ("禁用")
            w498 = FALSE ("可见")
            n496 = local write "公式显示"("") -> ()
            n497 = local write "时间计算标志"(TRUE ("布尔")) -> ()
            n498 = property on="扑克牌 1" class="Ring (严格)"("DisabledEnum"=w497) -> ()  [unwired: 2 in, 2 out]
            n499 = property on="扑克牌 2" class="Ring (严格)"("DisabledEnum"=w497) -> ()  [unwired: 2 in, 2 out]
            n500 = property on="扑克牌 3" class="Ring (严格)"("DisabledEnum"=w497) -> ()  [unwired: 2 in, 2 out]
            n501 = property on="扑克牌 4" class="Ring (严格)"("DisabledEnum"=w497) -> ()  [unwired: 2 in, 2 out]
            n502 = call "随机生成扑克牌.vi"() -> ("牌4值"=w488:dbl, "牌2值"=w490:dbl, "牌3值"=w489:dbl, "牌1值"=w491:dbl, "牌4"=w492:dbl, "牌3"=w493:dbl, "牌2"=w494:dbl, "牌1"=w495:dbl)
            n503 = call "计算主体.vi"("d"=w488, "c"=w489, "b"=w490, "a"=w491) -> ("算法总数"=w499:i32, "所有正解"=w500:string[])  [unwired: 1 in, 1 out]
            n504 = local write "牌值1"(w491) -> ()
            n505 = local write "牌值 2"(w490) -> ()
            n506 = local write "扑克牌 1"(w495) -> ()
            n507 = local write "扑克牌 2"(w494) -> ()
            n508 = property on="牌遮 1" class="TabCtl (严格)"("Visible"=w498) -> ()  [unwired: 2 in, 2 out]
            n509 = property on="牌遮 2" class="TabCtl (严格)"("Visible"=w498) -> ()  [unwired: 2 in, 2 out]
            n510 = property on="牌遮 3" class="TabCtl (严格)"("Visible"=w498) -> ()  [unwired: 2 in, 2 out]
            n511 = property on="牌遮 4" class="TabCtl (严格)"("Visible"=w498) -> ()  [unwired: 2 in, 2 out]
            n512 = local write "算法总数"(w499) -> ()
            n513 = local write "所有正解"(w500) -> ()
            n514 = local write "牌值 3"(w489) -> ()
            n515 = local write "牌值 4"(w488) -> ()
            n516 = local write "扑克牌 3"(w493) -> ()
            n517 = local write "扑克牌 4"(w492) -> ()
          }
          frame #1 {
            n518 = local write "新游戏标志"(FALSE ("新游戏标志")) -> ()
          }
        }
      }
    }
  }
  n519 = property on="开始游戏" class="Bool"("DisabledEnum"=T1."Enabled" ("禁用")) -> ()  [unwired: 2 in, 2 out]
  n520 = local write "所有正解"(string[] [] ("所有正解")) -> ()
  n521 = property on="牌遮 1" class="TabCtl (严格)"("Visible"=w20) -> ()  [unwired: 2 in, 2 out]
  n522 = property on="牌遮 2" class="TabCtl (严格)"("Visible"=w20) -> ()  [unwired: 2 in, 2 out]
  n523 = property on="牌遮 3" class="TabCtl (严格)"("Visible"=w20) -> ()  [unwired: 2 in, 2 out]
  n524 = property on="牌遮 4" class="TabCtl (严格)"("Visible"=w20) -> ()  [unwired: 2 in, 2 out]
  n525 = local write "扑克牌 1"(w22) -> ()
  n526 = local write "扑克牌 2"(w22) -> ()
  n527 = local write "扑克牌 3"(w22) -> ()
  n528 = local write "扑克牌 4"(w22) -> ()
  n529 = property on="扑克牌 1" class="Ring (严格)"("DisabledEnum"=w21) -> ()  [unwired: 2 in, 2 out]
  n530 = property on="扑克牌 2" class="Ring (严格)"("DisabledEnum"=w21) -> ()  [unwired: 2 in, 2 out]
  n531 = property on="扑克牌 3" class="Ring (严格)"("DisabledEnum"=w21) -> ()  [unwired: 2 in, 2 out]
  n532 = property on="扑克牌 4" class="Ring (严格)"("DisabledEnum"=w21) -> ()  [unwired: 2 in, 2 out]
  n533 = call <vilib>:"High Resolution Relative Seconds.vi"() -> ("relative seconds"=w12:dbl)
  n534 = local write "错题库"(dbl[][] [] ("错题库")) -> ()
  n535 = local write "time1"(w12) -> ()
  n536 = local write "表格"(string[][] [] ("表格")) -> ()
  n537 = local write "文件路径输入控件"(path "" ("文件路径输入控件")) -> ()
  n538 = while {
    stop <- FALSE stop-if-true
    n539 = case shown="真" "时间计算标志" {
      frame False {
      }
      frame True {
        n540 = local read "新游戏标志"() -> (w510:bool)
        "新游戏标志 2" <- w510
        n541 = call "已用时间"("Reset"=w510) -> ("Elapsed Time (s)"=w509:dbl)  [unwired: 11 in, 7 out]
        n542 = Number To Fractional String(number=w509, precision (6)=i16 2 ("精度(6)")) -> (F-format string=w507:string)  [unwired: 2 in]
        n543 = Concatenate Strings(w507, "s" ("字符串")) -> (→"已用时间":string)
      }
    }
  }
  n544 = local write "公式显示"("") -> ()
  n545 = local write "已用时间"("0.00s" ("连接的字符串")) -> ()
  n546 = local write "时间计算标志"(FALSE ("布尔")) -> ()
  n547 = local write "重做次数"(1 ("重做次数")) -> ()
  n548 = local write "游戏界面"(enum32{"主界面", "批量计算"}."主界面" ("选项卡控件")) -> ()
  n549 = local write "重做标志"(FALSE ("重做标志")) -> ()
  n550 = local write "新游戏标志"(FALSE ("新游戏标志")) -> ()
  "运算符输入次数" <- 0.0 ("运算符输入次数")
  "分数提示" <- "胜利/失败: 0/0" ("分数提示")
  "失败次数" <- w15
  "成功次数" <- w15
  "结果显示" <- "批量计算   组数据，有解率   %，共耗时   s。" ("字符串")
  "错题库" <- dbl[][] [] ("错题库")
  "有解次数" <- 0.0 ("无解次数")
